vi "stage_get_position.vi"(8 "error in (no error)":errorcluster, 10 "Stage Name":string, 11 "Stage in":refnum<class "Stage.lvclass">) -> (0 "error out":errorcluster, 2 "Position":dbl, 3 "Stage out":refnum<class "Stage.lvclass">)   [LabVIEW 2015, in "Stage.lvclass"]
uses:
  Stage.lvclass
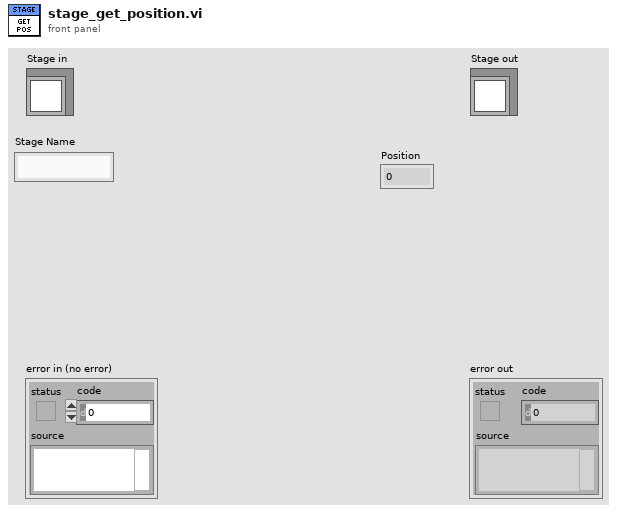
[diagram p1: front panel]
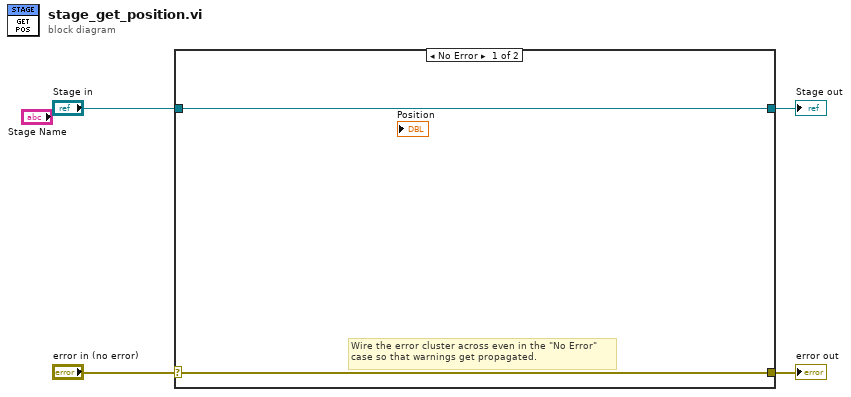
[diagram p0: block diagram]
diagram:
  n1 = case shown="No Error" "error in (no error)" {
    selector: "error in (no error)" -> [w5 w8]
    tunnel: [w5 w8] -> w3
    tunnel: [w6 w7] -> w1
    tunnel: "Stage in" -> [w6 w7]
    frame No Error {
      # "Wire the error cluster across even in the \"No Error\"\ncase so that warnings get propagated."
    }
    frame Error {
    }
  }
  "error out" <- w3
  "Stage out" <- w1
